vi "RunTestScenario.vi"(8 "error in (no error)":errorcluster, 11 "TestScenario in":refnum<class "TestScenario.lvclass">) -> (0 "error out":errorcluster, 3 "TestScenario out":refnum<class "TestScenario.lvclass">)   [LabVIEW 2015, in "TestScenario.lvclass"]
uses:
  TestScenario.lvclass
  ITestScenario.lvclass
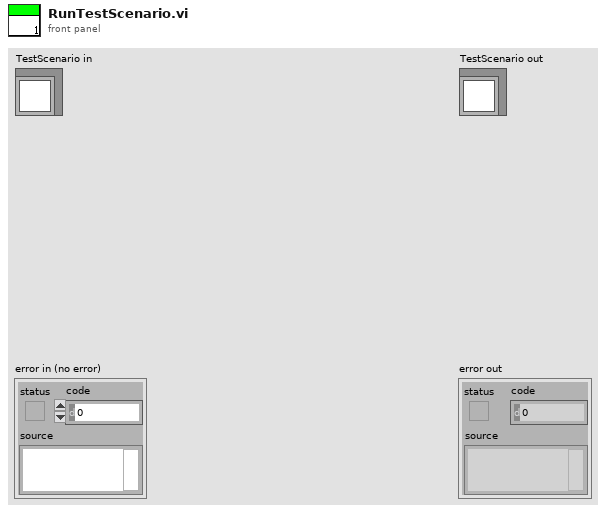
[diagram p1: front panel]
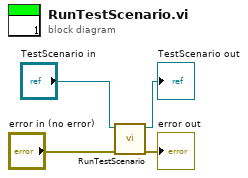
[diagram p0: block diagram]
diagram:
  n1 = call-parent "RunTestScenario.vi"("error in (no error)"="error in (no error)", "ITestScenario in"="TestScenario in") -> ("error out"=→"error out":errorcluster, "ITestScenario out"=→"TestScenario out":refnum<class "TestScenario.lvclass">)  [unwired: 8 in]
